vi "Read Notify Completion.vi"(8 "error in (no error)":errorcluster, 11 "Async Message in":refnum<class "Async Message.lvclass">) -> (0 "error out":errorcluster, 2 "Notify Completion":bool, 3 "Async Message out":refnum<class "Async Message.lvclass">)   [LabVIEW 2023, in "Async Methods Actor.lvlib" / "Async Message.lvclass"]
uses:
  Async Message.lvclass
  Async Message.lvclass/Async Message.ctl
  <vilib>/ActorFramework/Message Enqueuer/Message Enqueuer.lvclass
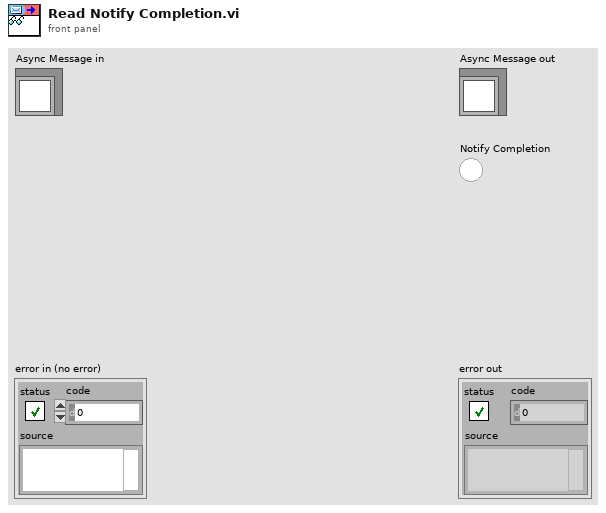
[diagram p1: front panel]
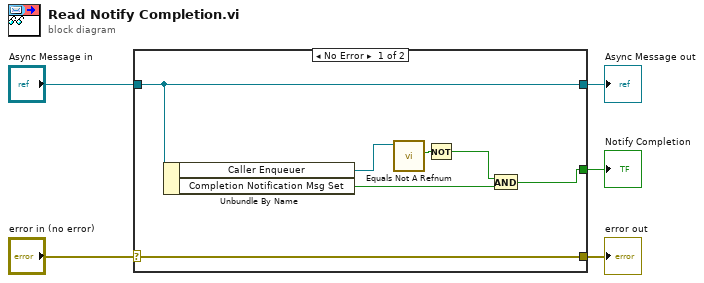
[diagram p0: block diagram]
diagram:
  n1 = case shown="No Error" "error in (no error)" {
    selector: "error in (no error)" -> [w12 w13]
    tunnel: [w12 w13] -> w4
    tunnel: [w11 w14] -> w2
    tunnel: "Async Message in" -> [w11 w14]
    tunnel: [w7 _] -> w1
    frame No Error {
      n2 = Unbundle By Name(w11) -> ("Caller Enqueuer"=w10:refnum<class "Message Enqueuer.lvclass">, "Completion Notification Msg Set"=w6:bool)
      n3 = call <vilib>:"Equals Not A Refnum.vi"("Message Enqueuer"=w10) -> ("Not a refnum?"=w9:bool)  [unwired: 10 in]
      n4 = Not(x=w9) -> (.not. x?=w8:bool)
      n5 = And(x=w8, y=w6) -> (x .and. y?=w7:bool)
    }
    frame Error {
    }
  }
  "error out" <- w4
  "Async Message out" <- w2
  "Notify Completion" <- w1
